vi "niDTS Calibration Cal Execute RF Test Initiate.vi"(0 "Template Tx Test Handle in":T1, 11 "error in (no error)":errorcluster) -> (4 "Template Tx Test Handle out":T1, 15 "error out":errorcluster)   [LabVIEW 2014, in "niDTS Utilities.lvlib"]
uses:
  niDTS Utilities.lvlib
  Includes/niDTS Calibration Cal Execute RF Test INC Handle.ctl
  Objects/BASE_class/niDTS Calibration Cal Execute RF Test.lvclass
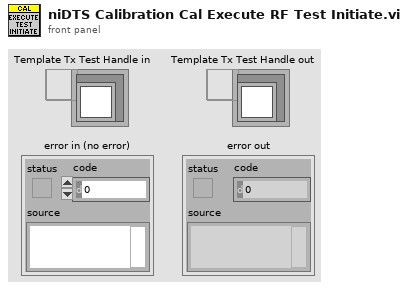
[diagram p1: front panel]
types:
  T1 = typedef "niDTS Utilities.lvlib/niDTS Calibration Cal Execute RF Test INC Handle.ctl" = refnum<data-value>
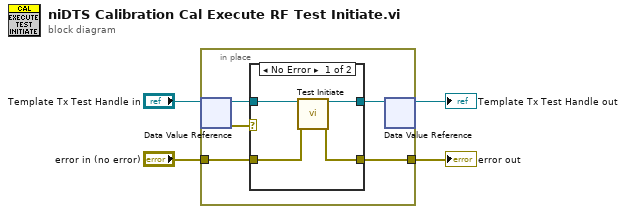
[diagram p0: block diagram]
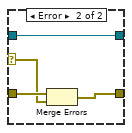
[diagram p2: hidden frame]
diagram:
  n1 = in-place {
    in-place-border: "error in (no error)" -> [w6]
    in-place-border: [w5] -> w1
    n2 = in-place-dvr #1("Template Tx Test Handle in") -> (w8:refnum<class "niDTS Calibration Cal Execute RF Test.lvclass">, w9:errorcluster)
    n3 = case shown="No Error" w9 {
      selector: w9 -> [_ w15]
      tunnel: w8 -> [w13 w17]
      tunnel: [w12 w17] -> w7
      tunnel: w6 -> [w11 w16]
      tunnel: [w10 w14] -> w5
      frame No Error {
        n4 = call-dynamic "Test Initiate.vi"("Template Tx Test in"=w13, "error in (no error)"=w11) -> ("Template Tx Test out"=w12:refnum<class "niDTS Calibration Cal Execute RF Test.lvclass">, "error out"=w10:errorcluster)  [unwired: 12 in]
      }
      frame Error {
        n5 = Merge Errors(w16, w15) -> (w14:errorcluster)
      }
    }
    n6 = in-place-dvr #1(w7) -> (→"Template Tx Test Handle out":T1)  [unwired: 1 out]
  }
  "error out" <- w1
